vi "DriveTeleop.vi"(6 "Quickturn":bool, 10 "Wheel":dbl(slide) scale=-1.0..1.0, 11 "Throttle":dbl format="%#_13g") -> ()   [LabVIEW 2017]
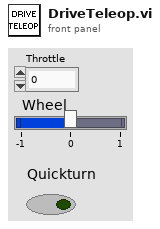
[diagram p1: front panel]
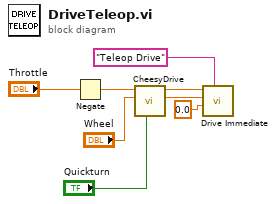
[diagram p0: block diagram]
diagram:
  n1 = Negate(x="Throttle") -> (-x=w4:dbl)
  n2 = call "CheesyDrive.vi"("Quickturn"="Quickturn", "Wheel"="Wheel", "Throttle"=w4) -> ("Right PWM"=w2:dbl, "Left PWM"=w3:dbl)  [unwired: 7 in]
  n3 = call "Drive Immediate.vi"("Description"="Teleop Drive", "Deadband Value"=0.0, "Right Setpoint"=w2, "Left Setpoint"=w3) -> ()  [unwired: 7 in, 1 out]
